vi "IMS Stepper Mover V2.vi"() -> ()   [LabVIEW 2018]
doc: "Use this template to build a producer/consumer design pattern with events to produce queue items. Use this design pattern instead of the User Interface Event Handler pattern for user interfaces when you want to execute code asynchronously in response to an event without slowing the user interface responsiveness."
uses:
  stepper motor state.ctl
  motor internal action.ctl
  slider setter action.ctl
  slider setter interal state.ctl
  stepper motor action.ctl
  publisher action.ctl
  slider action.ctl
panel:
  in  "Tab Control":enum32{"main", "init&stuff", "ignore"}(tab)
  in  "stepper state":T1=enum."stopped"
  in  "set angle":dbl(slide)=-18.244680851063833 scale=-95.0..95.0 scale format="%^#6_6g"
  in  "XY Graph":cluster{dbl[], dbl[]}[](graph)=[{[-0.2849184585575504, -0.22366098996767705, -0.16240352137780373, -0.10114605278793037, -0.03988858419805705, 0.02136888439181628, 0.08262635298168963, 0.14388382157156293, 0.20514129016143628, 0.2663987587513096, 0.32765622734118294, 0.3889136959310563, 0.45017116452092965, 0.511428633110803, 0.5726861017006762, 0.6339435702905496, 0.695201038880423, 0.7564585074702963, 0.8177159760601695, 0.878973444650043], [0.09392269147117449, 0.07372931280487197, 0.053535934138569455, 0.03334255547226694, 0.013149176805964419, -0.007044201860338106, -0.027237580526640617, -0.04743095919294313, -0.06762433785924565, -0.08781771652554818, -0.1080110951918507, -0.1282044738581532, -0.14839785252445573, -0.16859123119075825, -0.18878460985706075, -0.2089779885233633, -0.2291713671896658, -0.2493647458559683, -0.26955812452227085, -0.28975150318857334]}, {[0.02614672282429747, 0.020525177417073513, 0.014903632009849559, 0.0092820866026256, 0.003660541195401646, -0.0019610042118223085, -0.00758254961904627, -0.013204095026270225, -0.01882564043349418, -0.024447185840718134, -0.03006873124794209, -0.03569027665516605, -0.04131182206239001, -0.04693336746961396, -0.05255491287683792, -0.05817645828406187, -0.06379800369128583, -0.06941954909850978, -0.07504109450573374, -0.08066263991295769], [0.2988584094275236, 0.23460385140060602, 0.17034929337368845, 0.10609473534677089, 0.04184017731985329, -0.022414380707064308, -0.08666893873398185, -0.15092349676089944, -0.21517805478781704, -0.27943261281473464, -0.34368717084165223, -0.40794172886856983, -0.4721962868954873, -0.5364508449224049, -0.6007054029493225, -0.6649599609762401, -0.7292145190031577, -0.7934690770300753, -0.8577236350569929, -0.9219781930839105]}, {[1.0, 0.9980267284282716, 0.9921147013144779, 0.9822872507286887, 0.9685831611286311, 0.9510565162951535, 0.9297764858882513, 0.9048270524660195, 0.8763066800438636, 0.8443279255020151, 0.8090169943749475, 0.7705132427757891, 0.7289686274214116, 0.6845471059286886, 0.6374239897486896, 0.587785252292473, 0.5358267949789965, 0.48175367410171516, 0.42577929156507266, 0.36812455268467786, 0.30901699437494745, 0.24868988716485474, 0.18738131458572452, 0.12533323356430426, 0.0627905195293133, -1.6081428723391245e-16, -0.0627905195293134, -0.12533323356430437, -0.18738131458572482, -0.24868988716485485, -0.30901699437494756, -0.368124552684678, -0.4257792915650727, -0.48175367410171543, -0.5358267949789969, -0.587785252292473, -0.6374239897486897, -0.6845471059286887, -0.7289686274214117, -0.7705132427757894, -0.8090169943749473, -0.8443279255020151, -0.8763066800438636, -0.9048270524660196, -0.9297764858882515, -0.9510565162951536, -0.9685831611286311, -0.9822872507286887, -0.9921147013144779, -0.9980267284282716, -1.0, -0.9980267284282716, -0.9921147013144779, -0.9822872507286886, -0.9685831611286311, -0.9510565162951535, -0.9297764858882512, -0.9048270524660195, -0.8763066800438635, -0.844327925502015, -0.8090169943749472, -0.770513242775789, -0.7289686274214116, -0.6845471059286886, -0.6374239897486895, -0.5877852522924732, -0.5358267949789963, -0.48175367410171527, -0.42577929156507216, -0.3681245526846778, -0.30901699437494756, -0.24868988716485443, -0.18738131458572463, -0.12533323356430373, -0.06279051952931321, -1.836909530733566e-16, 0.06279051952931372, 0.12533323356430423, 0.18738131458572513, 0.24868988716485493, 0.30901699437494723, 0.36812455268467825, 0.4257792915650726, 0.4817536741017157, 0.5358267949789968, 0.5877852522924737, 0.63742398974869, 0.6845471059286886, 0.7289686274214119, 0.7705132427757894, 0.8090169943749478, 0.8443279255020153, 0.8763066800438636, 0.9048270524660197, 0.9297764858882515, 0.9510565162951538, 0.9685831611286312, 0.9822872507286887, 0.9921147013144779, 0.9980267284282716], [0.0, 0.06279051952931337, 0.12533323356430426, 0.18738131458572463, 0.2486898871648548, 0.3090169943749474, 0.368124552684678, 0.4257792915650727, 0.4817536741017153, 0.5358267949789967, 0.5877852522924731, 0.6374239897486897, 0.6845471059286887, 0.7289686274214116, 0.7705132427757893, 0.8090169943749475, 0.8443279255020151, 0.8763066800438637, 0.9048270524660196, 0.9297764858882515, 0.9510565162951535, 0.9685831611286311, 0.9822872507286887, 0.9921147013144779, 0.9980267284282716, 1.0, 0.9980267284282716, 0.9921147013144778, 0.9822872507286886, 0.9685831611286311, 0.9510565162951535, 0.9297764858882513, 0.9048270524660195, 0.8763066800438635, 0.844327925502015, 0.8090169943749475, 0.7705132427757893, 0.7289686274214114, 0.6845471059286885, 0.6374239897486895, 0.5877852522924732, 0.5358267949789967, 0.4817536741017152, 0.4257792915650725, 0.36812455268467775, 0.3090169943749471, 0.24868988716485482, 0.18738131458572457, 0.1253332335643041, 0.06279051952931314, -3.216285744678249e-16, -0.06279051952931335, -0.12533323356430429, -0.18738131458572477, -0.24868988716485502, -0.30901699437494773, -0.3681245526846783, -0.42577929156507266, -0.4817536741017154, -0.5358267949789968, -0.5877852522924734, -0.63742398974869, -0.6845471059286887, -0.7289686274214116, -0.7705132427757894, -0.8090169943749473, -0.8443279255020153, -0.8763066800438636, -0.9048270524660198, -0.9297764858882515, -0.9510565162951535, -0.9685831611286312, -0.9822872507286887, -0.9921147013144779, -0.9980267284282716, -1.0, -0.9980267284282716, -0.9921147013144779, -0.9822872507286886, -0.9685831611286311, -0.9510565162951536, -0.9297764858882512, -0.9048270524660196, -0.8763066800438634, -0.844327925502015, -0.809016994374947, -0.770513242775789, -0.7289686274214116, -0.6845471059286883, -0.6374239897486896, -0.5877852522924726, -0.5358267949789963, -0.4817536741017153, -0.4257792915650722, -0.36812455268467786, -0.3090169943749468, -0.2486898871648545, -0.18738131458572468, -0.1253332335643038, -0.06279051952931326]}, {[0.1, 0.09980267284282716, 0.0992114701314478, 0.09822872507286888, 0.09685831611286311, 0.09510565162951536, 0.09297764858882514, 0.09048270524660196, 0.08763066800438636, 0.08443279255020152, 0.08090169943749476, 0.07705132427757892, 0.07289686274214116, 0.06845471059286887, 0.06374239897486897, 0.05877852522924731, 0.05358267949789966, 0.04817536741017152, 0.042577929156507266, 0.03681245526846779, 0.030901699437494747, 0.024868988716485477, 0.018738131458572452, 0.012533323356430426, 0.006279051952931331, -1.6081428723391246e-17, -0.0062790519529313405, -0.012533323356430438, -0.018738131458572484, -0.024868988716485487, -0.030901699437494757, -0.0368124552684678, -0.04257792915650727, -0.048175367410171546, -0.05358267949789969, -0.05877852522924731, -0.06374239897486898, -0.06845471059286888, -0.07289686274214117, -0.07705132427757894, -0.08090169943749474, -0.08443279255020152, -0.08763066800438636, -0.09048270524660196, -0.09297764858882515, -0.09510565162951537, -0.09685831611286311, -0.09822872507286888, -0.0992114701314478, -0.09980267284282716, -0.1, -0.09980267284282716, -0.0992114701314478, -0.09822872507286887, -0.09685831611286311, -0.09510565162951536, -0.09297764858882512, -0.09048270524660196, -0.08763066800438635, -0.0844327925502015, -0.08090169943749473, -0.07705132427757891, -0.07289686274214116, -0.06845471059286887, -0.06374239897486896, -0.05877852522924733, -0.05358267949789963, -0.04817536741017153, -0.04257792915650722, -0.036812455268467784, -0.030901699437494757, -0.024868988716485445, -0.018738131458572463, -0.012533323356430374, -0.006279051952931321, -1.836909530733566e-17, 0.006279051952931373, 0.012533323356430424, 0.018738131458572515, 0.024868988716485494, 0.030901699437494726, 0.036812455268467825, 0.042577929156507266, 0.048175367410171574, 0.05358267949789968, 0.05877852522924737, 0.063742398974869, 0.06845471059286887, 0.07289686274214119, 0.07705132427757894, 0.08090169943749478, 0.08443279255020153, 0.08763066800438636, 0.09048270524660197, 0.09297764858882515, 0.09510565162951538, 0.09685831611286312, 0.09822872507286888, 0.0992114701314478, 0.09980267284282716], [0.0, 0.006279051952931338, 0.012533323356430426, 0.018738131458572463, 0.02486898871648548, 0.03090169943749474, 0.0368124552684678, 0.04257792915650727, 0.04817536741017153, 0.05358267949789967, 0.058778525229247314, 0.06374239897486898, 0.06845471059286888, 0.07289686274214116, 0.07705132427757894, 0.08090169943749476, 0.08443279255020152, 0.08763066800438638, 0.09048270524660196, 0.09297764858882515, 0.09510565162951536, 0.09685831611286311, 0.09822872507286888, 0.0992114701314478, 0.09980267284282716, 0.1, 0.09980267284282716, 0.09921147013144778, 0.09822872507286887, 0.09685831611286311, 0.09510565162951536, 0.09297764858882514, 0.09048270524660196, 0.08763066800438635, 0.0844327925502015, 0.08090169943749476, 0.07705132427757894, 0.07289686274214115, 0.06845471059286885, 0.06374239897486896, 0.05877852522924733, 0.05358267949789967, 0.048175367410171525, 0.04257792915650725, 0.03681245526846778, 0.030901699437494712, 0.024868988716485484, 0.01873813145857246, 0.01253332335643041, 0.0062790519529313145, -3.216285744678249e-17, -0.006279051952931335, -0.01253332335643043, -0.018738131458572477, -0.024868988716485504, -0.030901699437494774, -0.03681245526846783, -0.042577929156507266, -0.04817536741017154, -0.05358267949789968, -0.05877852522924734, -0.063742398974869, -0.06845471059286888, -0.07289686274214116, -0.07705132427757894, -0.08090169943749474, -0.08443279255020153, -0.08763066800438636, -0.09048270524660199, -0.09297764858882515, -0.09510565162951536, -0.09685831611286312, -0.09822872507286888, -0.0992114701314478, -0.09980267284282716, -0.1, -0.09980267284282716, -0.0992114701314478, -0.09822872507286887, -0.09685831611286311, -0.09510565162951537, -0.09297764858882512, -0.09048270524660196, -0.08763066800438635, -0.0844327925502015, -0.0809016994374947, -0.07705132427757891, -0.07289686274214116, -0.06845471059286883, -0.06374239897486897, -0.05877852522924726, -0.05358267949789963, -0.04817536741017153, -0.042577929156507224, -0.03681245526846779, -0.03090169943749468, -0.02486898871648545, -0.01873813145857247, -0.012533323356430379, -0.006279051952931327]}, {[0.0, 0.0, 0.0, 0.0, 0.0, 0.0, 0.0, 0.0, 0.0, 0.0, 0.0, 0.0, 0.0, 0.0, 0.0, 0.0, 0.0, 0.0, 0.0, 0.0], [1.1, 1.135, 1.1700000000000002, 1.205, 1.24, 1.2750000000000001, 1.31, 1.345, 1.3800000000000001, 1.415, 1.4500000000000002, 1.485, 1.52, 1.5550000000000002, 1.59, 1.625, 1.6600000000000001, 1.695, 1.73, 1.7650000000000001]}, {[6.735334946023075e-17, 6.796565263714194e-17, 6.857795581405312e-17, 6.919025899096432e-17, 6.980256216787551e-17, 7.04148653447867e-17, 7.102716852169788e-17, 7.163947169860908e-17, 7.225177487552027e-17, 7.286407805243145e-17, 7.347638122934264e-17, 7.408868440625383e-17, 7.470098758316503e-17, 7.53132907600762e-17, 7.59255939369874e-17, 7.653789711389858e-17, 7.715020029080977e-17, 7.776250346772096e-17, 7.837480664463216e-17, 7.898710982154334e-17], [1.1, 1.11, 1.12, 1.1300000000000001, 1.1400000000000001, 1.1500000000000001, 1.1600000000000001, 1.1700000000000002, 1.1800000000000002, 1.1900000000000002, 1.2000000000000002, 1.21, 1.22, 1.23, 1.24, 1.25, 1.26, 1.27, 1.28, 1.29]}, {[-0.09587131702242406, -0.09674287444990064, -0.09761443187737723, -0.0984859893048538, -0.0993575467323304, -0.10022910415980697, -0.10110066158728355, -0.10197221901476014, -0.10284377644223672, -0.10371533386971331, -0.10458689129718989, -0.10545844872466646, -0.10633000615214305, -0.10720156357961963, -0.10807312100709622, -0.1089446784345728, -0.10981623586204937, -0.11068779328952597, -0.11155935071700254, -0.11243090814447912], [-1.0958141679009201, -1.1057761148818375, -1.115738061862755, -1.1257000088436726, -1.13566195582459, -1.1456239028055073, -1.1555858497864249, -1.1655477967673424, -1.1755097437482598, -1.1854716907291771, -1.1954336377100947, -1.2053955846910123, -1.2153575316719296, -1.225319478652847, -1.2352814256337645, -1.245243372614682, -1.2552053195955994, -1.2651672665765168, -1.2751292135574344, -1.285091160538352]}]
  out "cur angle":dbl(slide)=-95.0 scale=-95.0..95.0 scale format="%^#6_6g"
  in  "set step !":dbl(slide)=6845.744680851064 min=0.0 max=16000.0 scale=0.0..16500.0 scale format="%^#6_6g"
  out "cur step":dbl(slide) scale=0.0..16500.0
  in  "Go!":bool
  in  "Stop!":bool
  in  "set speed!":i32=2500
  out "Moving..":bool
  out "error out":errorcluster
  out "Current Bottom Position":dbl format="%.4f"
  in  "Move to Bottom Position (deg or in)":dbl=95.83933701824397 format="%.4f"
  in  "Rotator":T2(ring)=enum."System B 50 mm Magnet"
  out "Timeout error":bool
  in  "Exit!":bool
  in  "Instrument Address":refnum<visa-resource-name>="ASRL2::INSTR"
  in  "Set to zero!":bool
  in  "Init!":bool
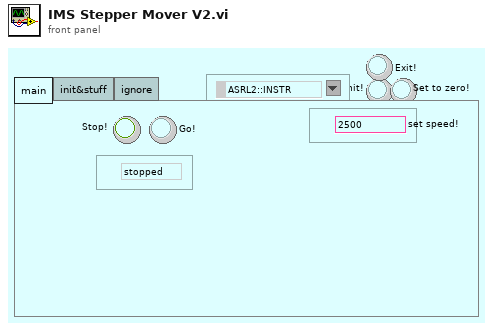
[diagram p1: front panel]
types:
  T1 = typedef "stepper motor state.ctl" = enum16{"moving", "stopped"}
  T2 = enum16{"Dilution Fridge SCM 1", "System A SCM 2", "System B 50 mm Magnet", "He-3 32 mm Magnet", "Portable Dil Fridge Rotator", "Linear Position", "System E Probe 1"}
  T3 = typedef "stepper motor action.ctl" = enum16{"go", "void", "stop", "check", "init", "sync", "set", "set speed"}
  T4 = typedef "slider setter interal state.ctl" = cluster{"set pos slider":refnum<vi>, "cur angle slider":refnum<vi>, "current pos... slider":refnum<vi>, "XY Graph":refnum<vi>, "set angle":dbl, "pos angle":dbl, "set angle slider":refnum<vi>}
  T5 = typedef "slider setter action.ctl" = enum16{"--update circle", "set step slider moves", "cursor moves", "current pos changed", "init", "void", "--draw current lie", "--draw set line", "--move current step slider", "--move set step slider", "--draw limit lines", "check", "--move set angle slider", "--move current angle slider", "set angle slider moves", "--move cursor", "set set step", "set current step"}
  T6 = typedef "motor internal action.ctl" = enum16{"set slider moves", "update scale", "exit", "current positon changed"}
  T7 = typedef "slider action.ctl" = enum16{"check", "copy range", "set from value", "set from ratio", "set from slider", "read using other slider"}
  T8 = typedef "publisher action.ctl" = enum16{"set", "get"}
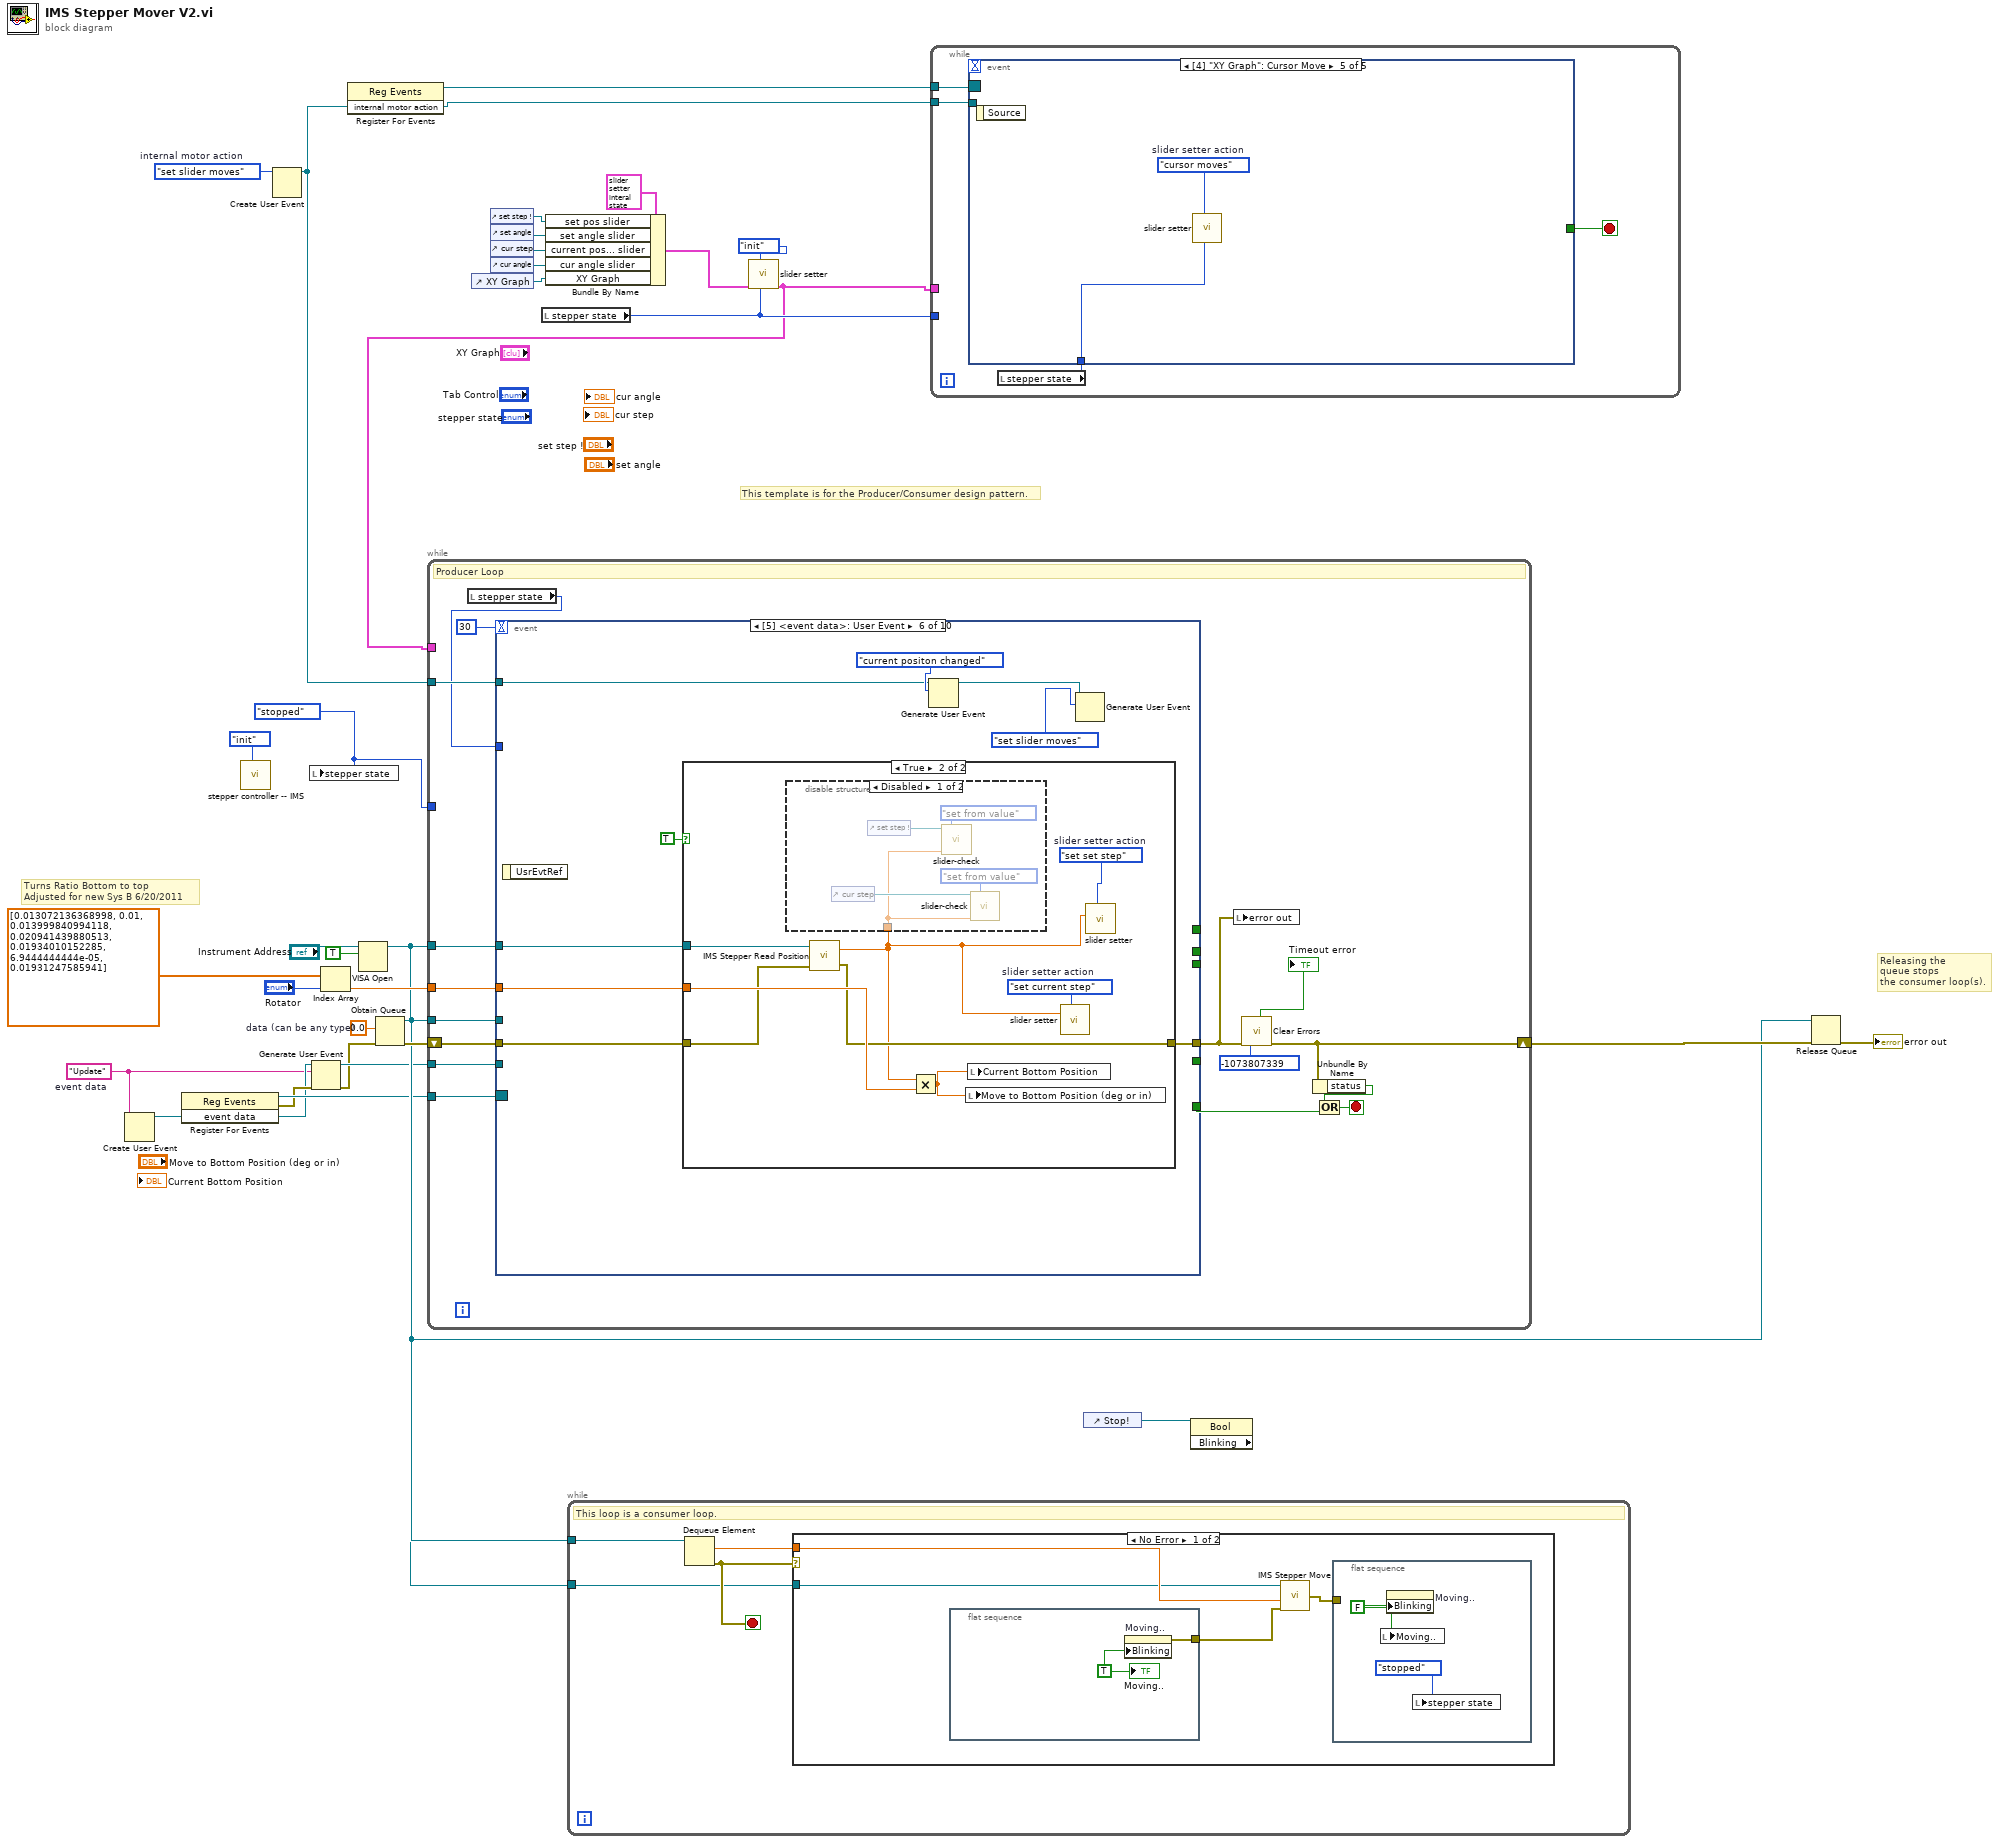
[diagram p0: block diagram]
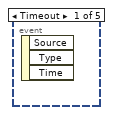
[diagram p2: hidden frame]
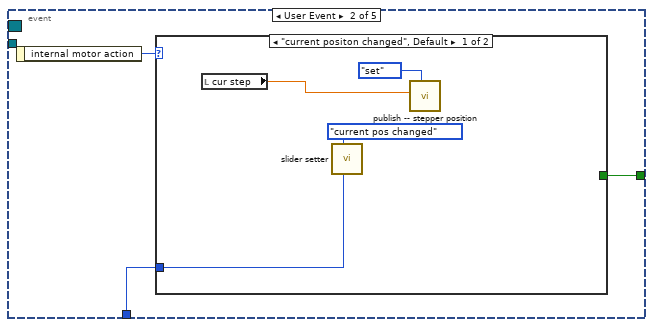
[diagram p3: hidden frame]
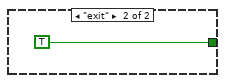
[diagram p4: hidden frame]
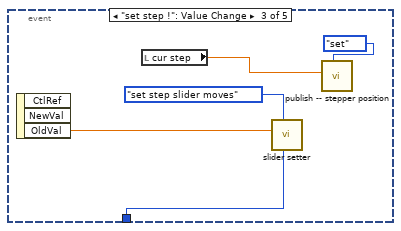
[diagram p5: hidden frame]
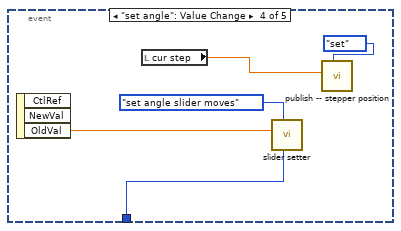
[diagram p6: hidden frame]
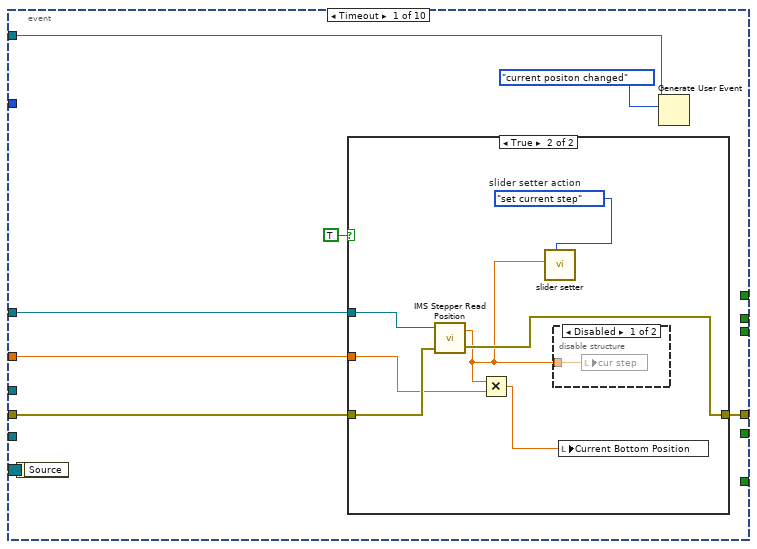
[diagram p8: hidden frame]
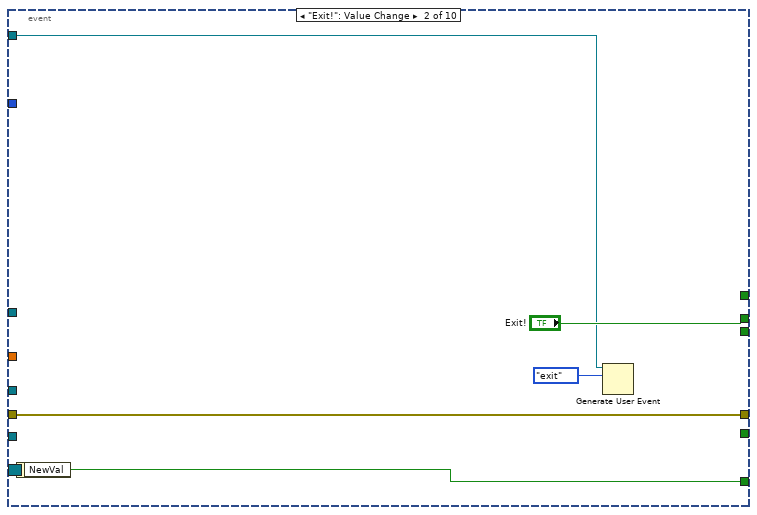
[diagram p11: hidden frame]
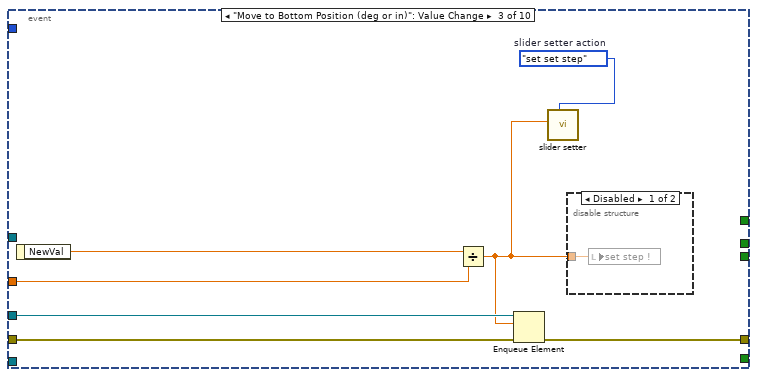
[diagram p12: hidden frame]
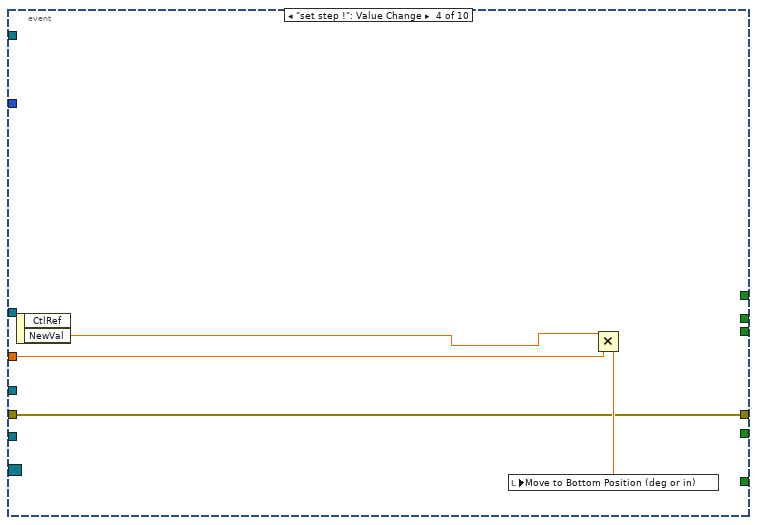
[diagram p14: hidden frame]
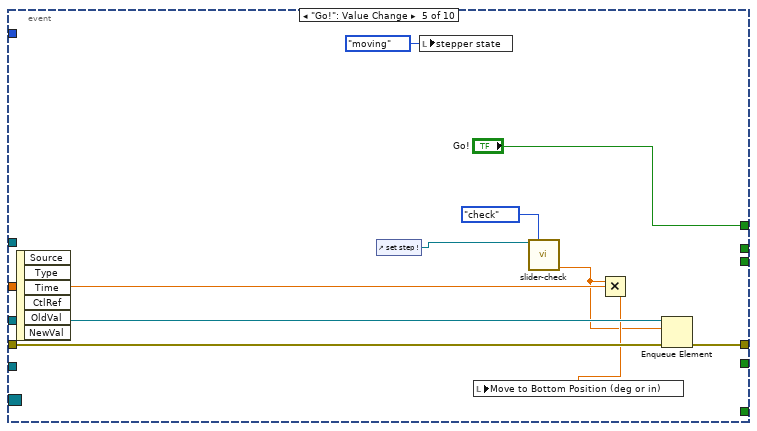
[diagram p15: hidden frame]
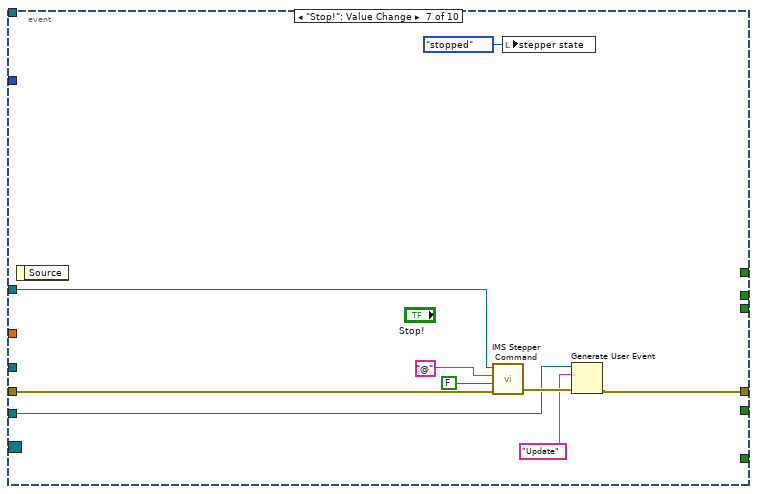
[diagram p18: hidden frame]
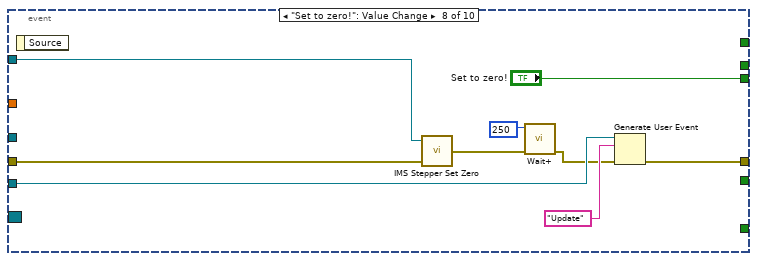
[diagram p19: hidden frame]
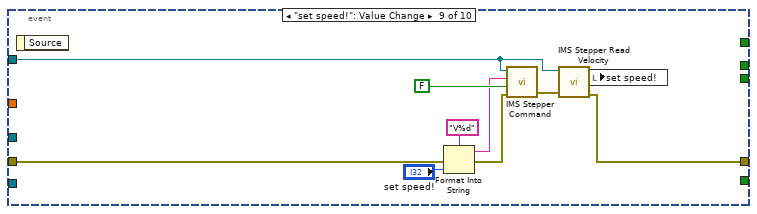
[diagram p20: hidden frame]
diagram:
  w2 = stepper_motor_state."stopped" ("stepper state")
  w15 = motor_internal_action."set slider moves"  # internal motor action
  w18 = "Update"  # event data
  w31 = 0.0  # data (can be any type)
  # "Turns Ratio Bottom to top\nAdjusted for new Sys B 6/20/2011"
  # "Releasing the\nqueue stops\nthe consumer loop(s)."
  # "This template is for the Producer/Consumer design pattern."
  n1 = Create User Event(user event datatype=w18) -> (user event=w21:refnum<user-event>)  [unwired: 1 in, 1 out]
  n2 = register-events(w21) -> (reference out=w23:refnum<event-registration>, error out=w22:errorcluster)  [unwired: 2 in]
  n3 = call "stepper controller -- IMS.vi"("stepper motor action"=stepper_motor_action."init") -> ()  [unwired: 10 in, 1 out]
  n4 = Create User Event(user event datatype=w15) -> (user event=w12:refnum<user-event>)  [unwired: 1 in, 1 out]
  n5 = local write "stepper state"(w2) -> ()
  n6 = Generate User Event(user event=w21, event data cluster=w18, error in=w22) -> (user event out=w20:refnum<user-event>, error out=w19:errorcluster)  [unwired: 1 in]
  n7 = Index Array(array=dbl[] [0.013072136368998, 0.01, 0.013999840994118, 0.020941439880513, 0.01934010152285, 6.9444444444e-05, 0.01931247585941], index="Rotator") -> (element=w25:dbl)
  n8 = register-events(w12) -> (reference out=w16:refnum<event-registration>)  [unwired: 2 in, 1 out]
  n9 = VISA Open(duplicate session (F)=TRUE, VISA resource name="Instrument Address") -> (VISA resource name=w24:refnum<visa-resource-name>)  [unwired: 3 in, 1 out]
  n10 = Obtain Queue(element data type=w31, error in (no error)=w19) -> (queue out=w30:refnum<queue>, error out=w33:errorcluster)  [unwired: 3 in, 1 out]
  n11 = control-ref of="XY Graph"() -> (w10:refnum<vi>)
  n12 = control-ref of="set step !"() -> (w6:refnum<vi>)
  n13 = control-ref of="set angle"() -> (w7:refnum<vi>)
  n14 = control-ref of="cur step"() -> (w8:refnum<vi>)
  n15 = control-ref of="cur angle"() -> (w9:refnum<vi>)
  n16 = local read "stepper state"() -> (w13:T1)
  n17 = Bundle By Name(cluster=T4 {"set pos slider"=refnum, "cur angle slider"=refnum, "current pos... slider"=refnum, "XY Graph"=refnum, "set angle"=0.0, "pos angle"=0.0, "set angle slider"=refnum} ("Cluster"), "set pos slider"=w6, "set angle slider"=w7, "current pos... slider"=w8, "cur angle slider"=w9, "XY Graph"=w10) -> (w5:T4)
  n18 = while {
    tunnel: w30 -> [w37]
    tunnel: w24 -> [w34]
    stop <- w36 stop-if-true
    # "This loop is a consumer loop."
    n19 = Dequeue Element(queue=w37) -> (element=w35:dbl, error out=w36:errorcluster)  [unwired: 2 in, 2 out]
    n20 = case shown="No Error" w36 {
      tunnel: w35 -> [w41 _]
      tunnel: w34 -> [w40 _]
      frame No Error {
        n21 = flat-sequence {
          tunnel: [w42] -> w39
          frame #0 {
            w43 = TRUE ("Moving")
            n22 = property on="Moving.." class="Bool (strict)"("Blinking"=w43) -> (error out=w42:errorcluster)  [unwired: 2 in, 1 out]
            "Moving.." <- w43
          }
        }
        n23 = call "IMS Stepper Move.vi"("Instrument Address"=w40, "Distance"=w41, "error in (no error)"=w39) -> ("error out"=w38:errorcluster)  [unwired: 2 in]
        n24 = flat-sequence {
          tunnel: w38 -> [_]
          frame #0 {
            w45 = FALSE ("Moving")
            n25 = local write "Moving.."(w45) -> ()
            n26 = property on="Moving.." class="Bool (strict)"("Blinking"=w45) -> ()  [unwired: 2 in, 2 out]
            n27 = local write "stepper state"(stepper_motor_state."stopped" ("stepper state")) -> ()
          }
        }
      }
      frame Error {
      }
    }
  }
  n28 = call "slider setter.vi"("stepper motor state"=w13, "slider setter action"=slider_setter_action."init", "state in"=w5) -> ("state OUT"=w3:T4)  [unwired: 8 in]
  n29 = while {
    shift-right: [w49] -> w32
    shift-left: w33 -> [w60]
    tunnel: w30 -> [w61]
    tunnel: w24 -> [w55]
    tunnel: w25 -> [w54]
    tunnel: w23 -> [w53]
    tunnel: w20 -> [w52]
    tunnel: w12 -> [w47]
    tunnel: w3 -> [_]
    tunnel: w2 -> [_]
    stop <- w58 stop-if-true
    # "Producer Loop"
    n30 = local read "stepper state"() -> (w46:T1)
    n31 = event shown="[5] <event data>: User Event" {
      selector: w53 -> [_ _ _ _ _ _ _ _ _ _]
      dyn-events: _ -> [_ _ _ _ _ _ _ _ _ _]
      timeout: 30 -> [_ _ _ _ _ _ _ _ _ _]
      tunnel: w61 -> [_ _ w89 _ w105 _ _ _ _ _]
      tunnel: w60 -> [w68 w82 w88 w93 w104 w112 w135 w146 w152 w165]
      tunnel: [w63 w82 w87 w93 w103 w109 w133 w144 w147 w168] -> w48
      tunnel: [_ w81 _ _ _ _ _ _ _ _] -> w59
      tunnel: w55 -> [w67 _ _ _ _ w113 w137 w145 w149 w162]
      tunnel: w54 -> [w66 _ w86 w95 w102 w114 _ _ _ _]
      tunnel: w52 -> [_ _ _ _ _ _ w131 w143 _ w167]
      tunnel: [_ _ _ _ _ _ _ "Set to zero!" _ _] -> _
      tunnel: [_ _ _ _ _ _ _ _ _ "Init!"] -> _
      tunnel: [_ "Exit!" _ _ _ _ _ _ _ _] -> _
      tunnel: w47 -> [w65 w78 _ w92 _ w110 _ _ _ _]
      tunnel: [_ _ _ _ "Go!" _ _ _ _ _] -> _
      tunnel: [_ _ _ w92 _ _ _ _ _ _] -> _
      tunnel: w46 -> [_ _ _ _ _ _ _ _ _ _]
      event Timeout {
        n32 = event-data() -> ()  [unwired: 1 in, 1 out]
        n33 = case shown="True" TRUE {
          tunnel: w68 -> [w69 w76]
          tunnel: w67 -> [_ w75]
          tunnel: w66 -> [_ w74]
          tunnel: [w69 w72] -> w63
          frame False {
          }
          frame True {
            w70 = slider_setter_action."set current step"  # slider setter action
            n34 = call "IMS Stepper Read Position.vi"("error in (no error)"=w76, "Instrument Address"=w75) -> ("error out"=w72:errorcluster, "Response"=w71:dbl)  [unwired: 1 in]
            n35 = Multiply(x=w71, y=w74) -> (x*y=w73:dbl)
            n36 = call "slider setter.vi"("slider setter action"=w70, "value"=w71) -> ()  [unwired: 9 in, 1 out]
            n37 = disable-structure shown="Disabled" {
              disable-tunnel: w71 -> [w77 _]
              frame Disabled {
                n38 = local write "cur step"(w77) -> ()
              }
              frame Enabled {
              }
            }
            n39 = local write "Current Bottom Position"(w73) -> ()
          }
        }
        n40 = Generate User Event(user event=w65, event data cluster=motor_internal_action."current positon changed" ("event data")) -> ()  [unwired: 2 in, 2 out]
      }
      event "Exit!": Value Change {
        n41 = event-data() -> ("NewVal"=w81:bool)  [unwired: 1 in]
        n42 = Generate User Event(user event=w78, event data cluster=motor_internal_action."exit" ("event data")) -> ()  [unwired: 2 in, 2 out]
      }
      event "Move to Bottom Position (deg or in)": Value Change {
        w83 = slider_setter_action."set set step"  # slider setter action
        n43 = event-data() -> ("NewVal"=w85:dbl)  [unwired: 1 in]
        n44 = Divide(x=w85, y=w86) -> (x/y=w84:dbl)
        n45 = Enqueue Element(queue=w89, element=w84, error in (no error)=w88) -> (error out=w87:errorcluster)  [unwired: 1 in, 2 out]
        n46 = call "slider setter.vi"("slider setter action"=w83, "value"=w84) -> ()  [unwired: 9 in, 1 out]
        n47 = disable-structure shown="Disabled" {
          disable-tunnel: w84 -> [w90 _]
          frame Disabled {
            n48 = local write "set step !"(w90) -> ()
          }
          frame Enabled {
          }
        }
      }
      event "set step !": Value Change {
        n49 = event-data() -> ("NewVal"=w91:dbl)  [unwired: 1 in, 1 out]
        n50 = Multiply(x=w91, y=w95) -> (x*y=w94:dbl)
        n51 = local write "Move to Bottom Position (deg or in)"(w94) -> ()
      }
      event "Go!": Value Change {
        n52 = event-data() -> ()  [unwired: 1 in, 6 out]
        n53 = control-ref of="set step !"() -> (w97:refnum<vi>)
        n54 = local write "stepper state"(stepper_motor_state."moving" ("stepper state")) -> ()
        n55 = call "slider-check.vi"("slider"=w97, "slider action"=slider_action."check") -> ("value OUT"=w99:dbl)  [unwired: 9 in, 4 out]
        n56 = Multiply(x=w99, y=w102) -> (x*y=w101:dbl)
        n57 = local write "Move to Bottom Position (deg or in)"(w101) -> ()
        n58 = Enqueue Element(queue=w105, element=w99, error in (no error)=w104) -> (error out=w103:errorcluster)  [unwired: 1 in, 2 out]
      }
      event User Event {
        n59 = event-data() -> ()  [unwired: 1 in, 1 out]
        n60 = case shown="True" TRUE {
          tunnel: w114 -> [_ w123]
          tunnel: w113 -> [_ w122]
          tunnel: w112 -> [w115 w121]
          tunnel: [w115 w119] -> w109
          frame False {
          }
          frame True {
            w117 = slider_setter_action."set current step"  # slider setter action
            w118 = slider_setter_action."set set step"  # slider setter action
            n61 = call "IMS Stepper Read Position.vi"("error in (no error)"=w121, "Instrument Address"=w122) -> ("error out"=w119:errorcluster, "Response"=w116:dbl)  [unwired: 1 in]
            n62 = disable-structure shown="Disabled" {
              disable-tunnel: w116 -> [w124 _]
              frame Disabled {
                n63 = control-ref of="cur step"() -> (w127:refnum<vi>)
                n64 = control-ref of="set step !"() -> (w128:refnum<vi>)
                n65 = call "slider-check.vi"("slider"=w128, "slider action"=slider_action."set from value", "value IN"=w124) -> ()  [unwired: 8 in, 5 out]
                n66 = call "slider-check.vi"("slider"=w127, "slider action"=slider_action."set from value", "value IN"=w124) -> ()  [unwired: 8 in, 5 out]
              }
              frame Enabled {
              }
            }
            n67 = Multiply(x=w116, y=w123) -> (x*y=w120:dbl)
            n68 = local write "Move to Bottom Position (deg or in)"(w120) -> ()
            n69 = local write "Current Bottom Position"(w120) -> ()
            n70 = call "slider setter.vi"("slider setter action"=w117, "value"=w116) -> ()  [unwired: 9 in, 1 out]
            n71 = call "slider setter.vi"("slider setter action"=w118, "value"=w116) -> ()  [unwired: 9 in, 1 out]
          }
        }
        n72 = Generate User Event(user event=w110, event data cluster=motor_internal_action."current positon changed" ("event data")) -> (user event out=w108:refnum<user-event>)  [unwired: 2 in, 1 out]
        n73 = Generate User Event(user event=w108, event data cluster=motor_internal_action."set slider moves" ("event data")) -> ()  [unwired: 2 in, 2 out]
      }
      event "Stop!": Value Change {
        n74 = event-data() -> ()  [unwired: 1 in, 1 out]
        n75 = call "IMS Stepper Command.vi"("Instrument Address"=w137, "Command"="@", "Mode"=FALSE, "error in (no error)"=w135) -> ("error out"=w132:errorcluster)  [unwired: 2 in, 2 out]
        n76 = local write "stepper state"(stepper_motor_state."stopped" ("stepper state")) -> ()
        n77 = Generate User Event(user event=w131, event data cluster="Update" ("event data"), error in=w132) -> (error out=w133:errorcluster)  [unwired: 1 in, 1 out]
      }
      event "Set to zero!": Value Change {
        n78 = event-data() -> ()  [unwired: 1 in, 1 out]
        n79 = call "IMS Stepper Set Zero.vi"("error in (no error)"=w146, "Instrument Address"=w145) -> ("error out"=w140:errorcluster)  [unwired: 1 in]
        n80 = call "Wait+.vi"("Error In"=w140, "milliseconds to wait"=u32 250) -> ("Error Out"=w139:errorcluster)  [unwired: 4 in, 1 out]
        n81 = Generate User Event(user event=w143, event data cluster="Update" ("event data"), error in=w139) -> (error out=w144:errorcluster)  [unwired: 1 in, 1 out]
      }
      event "set speed!": Value Change {
        n82 = event-data() -> ()  [unwired: 1 in, 1 out]
        n83 = Format Into String(format string="V%d", error in=w152, "set speed!") -> (resulting string=w153:string, error out=w151:errorcluster)  [unwired: 1 in]
        n84 = call "IMS Stepper Command.vi"("Instrument Address"=w149, "Command"=w153, "Mode"=FALSE, "error in (no error)"=w151) -> ("error out"=w150:errorcluster)  [unwired: 2 in, 2 out]
        n85 = call "IMS Stepper Read Velocity.vi"("error in (no error)"=w150, "Instrument Address"=w149) -> ("error out"=w147:errorcluster, "Velocity"=w148:i32)  [unwired: 3 in, 1 out]
        n86 = local write "set speed!"(w148) -> ()
      }
      event "Init!": Value Change {
        n87 = event-data() -> ()  [unwired: 1 in, 1 out]
        n88 = call "IMS Stepper Init.vi"("error in (no error)"=w165, "Baud Rate"=u32 9600, "Instrument Address"=w162) -> ("error out"=w159:errorcluster)  [unwired: 1 in, 1 out]
        n89 = call "Wait+.vi"("Error In"=w159, "milliseconds to wait"=u32 250) -> ("Error Out"=w160:errorcluster)  [unwired: 4 in, 1 out]
        n90 = call "IMS Stepper Read Velocity.vi"("error in (no error)"=w160, "Instrument Address"=w162) -> ("error out"=w163:errorcluster, "Velocity"=w161:i32)  [unwired: 3 in, 1 out]
        n91 = local write "set speed!"(w161) -> ()
        n92 = Generate User Event(user event=w167, event data cluster="Update" ("event data"), error in=w163) -> (error out=w168:errorcluster)  [unwired: 1 in, 1 out]
      }
    }
    n93 = local write "error out"(w48) -> ()
    n94 = call <vilib>:"Clear Errors.vi"("error in (no error)"=w48, "specific error code to clear (0: all)"=-1073807339) -> ("error out"=w49:errorcluster, "specific error cleared?"=→"Timeout error":bool)  [unwired: 4 in]
    n95 = Unbundle By Name(w49) -> ("status"=w57:bool)
    n96 = Or(x=w57, y=w59) -> (x .or. y?=w58:bool)
  }
  n97 = while {
    tunnel: w16 -> [w172]
    tunnel: w13 -> [_]
    tunnel: w12 -> [w170]
    tunnel: w3 -> [_]
    stop <- w171 stop-if-true
    n98 = local read "stepper state"() -> (w169:T1)
    n99 = event shown="[4] \"XY Graph\": Cursor Move" {
      selector: w172 -> [_ _ _ _ _]
      dyn-events: _ -> [_ _ _ _ _]
      timeout: _ -> [_ _ _ _ _]
      tunnel: [_ w174 _ _ _] -> w171
      tunnel: w170 -> [_ _ _ _ _]
      tunnel: w169 -> [_ w173 w181 w186 w191]
      event Timeout {
        n100 = event-data() -> ()  [unwired: 1 in, 3 out]
      }
      event User Event {
        n101 = event-data() -> ("internal motor action"=w175:T6)  [unwired: 1 in]
        n102 = case shown="\"current positon changed\", Default" w175 {
          tunnel: [_ TRUE] -> w174
          tunnel: w173 -> [w176 _]
          frame "current positon changed", Default {
            n103 = local read "cur step"() -> (w178:dbl)
            n104 = call "slider setter.vi"("stepper motor state"=w176, "slider setter action"=slider_setter_action."current pos changed") -> ()  [unwired: 9 in, 1 out]
            n105 = call "publish -- stepper position.vi"("publisher action"=publisher_action."set", "stepper pos IN"=w178) -> ()  [unwired: 9 in, 1 out]
          }
          frame "exit" {
          }
        }
      }
      event "set step !": Value Change {
        n106 = event-data() -> ("OldVal"=w183:dbl)  [unwired: 1 in, 2 out]
        n107 = local read "cur step"() -> (w185:dbl)
        n108 = call "slider setter.vi"("stepper motor state"=w181, "slider setter action"=slider_setter_action."set step slider moves", "value"=w183) -> ()  [unwired: 8 in, 1 out]
        n109 = call "publish -- stepper position.vi"("publisher action"=publisher_action."set", "stepper pos IN"=w185) -> ()  [unwired: 9 in, 1 out]
      }
      event "set angle": Value Change {
        n110 = event-data() -> ("OldVal"=w188:dbl)  [unwired: 1 in, 2 out]
        n111 = local read "cur step"() -> (w190:dbl)
        n112 = call "slider setter.vi"("stepper motor state"=w186, "slider setter action"=slider_setter_action."set angle slider moves", "value"=w188) -> ()  [unwired: 8 in, 1 out]
        n113 = call "publish -- stepper position.vi"("publisher action"=publisher_action."set", "stepper pos IN"=w190) -> ()  [unwired: 9 in, 1 out]
      }
      event "XY Graph": Cursor Move {
        w192 = slider_setter_action."cursor moves"  # slider setter action
        n114 = event-data() -> ()  [unwired: 1 in, 1 out]
        n115 = call "slider setter.vi"("stepper motor state"=w191, "slider setter action"=w192) -> ()  [unwired: 9 in, 1 out]
      }
    }
  }
  n116 = control-ref of="Stop!"() -> (w1:refnum<vi>)
  n117 = property class="Bool" props=["Blinking"](reference=w1) -> ()  [unwired: 1 in, 3 out]
  n118 = Release Queue(queue=w30, error in (no error)=w32) -> (error out=→"error out":errorcluster)  [unwired: 1 in, 2 out]
